vi "array-add-element.vi"() -> ()   [LabVIEW 2014]
panel:
  in  "Data to extract":enum16{"All", "None", "Even ", "Odd"}(ring)
  out "Output Array":i32[](array[numeric])
  in  "Input Array":i32[](array[numeric])=[1, 2, 3, 4, 5, 6, 7, 8, 9, 10]
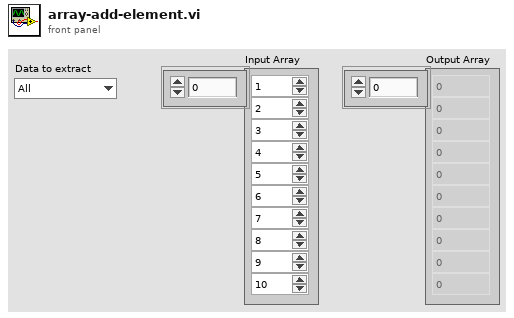
[diagram p1: front panel]
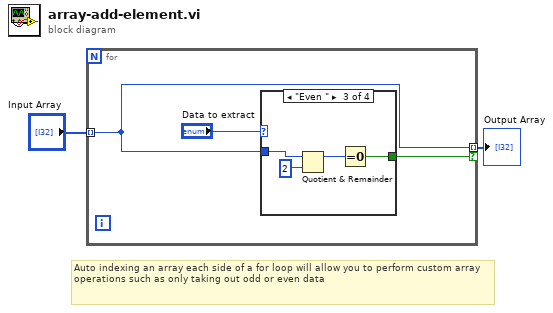
[diagram p0: block diagram]
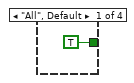
[diagram p2: hidden frame]
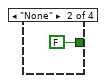
[diagram p3: hidden frame]
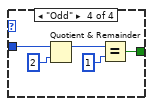
[diagram p4: hidden frame]
diagram:
  # "Auto indexing an array each side of a for loop will allow you to perform custom array operations such as only taking out odd or even data"
  n1 = for {
    tunnel: [w3] -> w2 mode=indexing if=w5
    tunnel: "Input Array" -> [w3] mode=indexing
    n2 = case shown="\"Even \"" "Data to extract" {
      tunnel: [TRUE FALSE w9 w12] -> w5
      tunnel: w3 -> [_ _ w8 w15]
      frame "All", Default {
      }
      frame "None" {
      }
      frame "Even " {
        n3 = Quotient & Remainder(x=w8, y=2) -> (x-y*floor(x/y)=w10:i32)  [unwired: 1 out]
        n4 = Equal To 0?(x=w10) -> (x = 0?=w9:bool)
      }
      frame "Odd" {
        n5 = Quotient & Remainder(x=w15, y=2) -> (x-y*floor(x/y)=w14:i32)  [unwired: 1 out]
        n6 = Equal?(x=w14, y=1) -> (x = y?=w12:bool)
      }
    }
  }
  "Output Array" <- w2
